vi "Array Parameter Size.vi"() -> ()   [LabVIEW 2020]
uses:
  868a90fa-e97d-4ae1-b623-939be4d37f0a.vi
  d44bdd64-d287-4cd4-98fd-2ffcf2f89dc6.vi
  <userlib>/_NEVSTOP/Communicable State Machine(CSM)/addons/MassData-Parameter/_support/FGV-MassData.vi
  <userlib>/_NEVSTOP/Communicable State Machine(CSM)/addons/MassData-Parameter/CSM MassData Parameter Support.lvlib
panel:
  out "Argument":string
  out "DBL":i32[](array[numeric])
  out "inside 2":i32
  out "inside":i32
  out "outside":i32
  out "unit (ms)":dbl[][](graph)
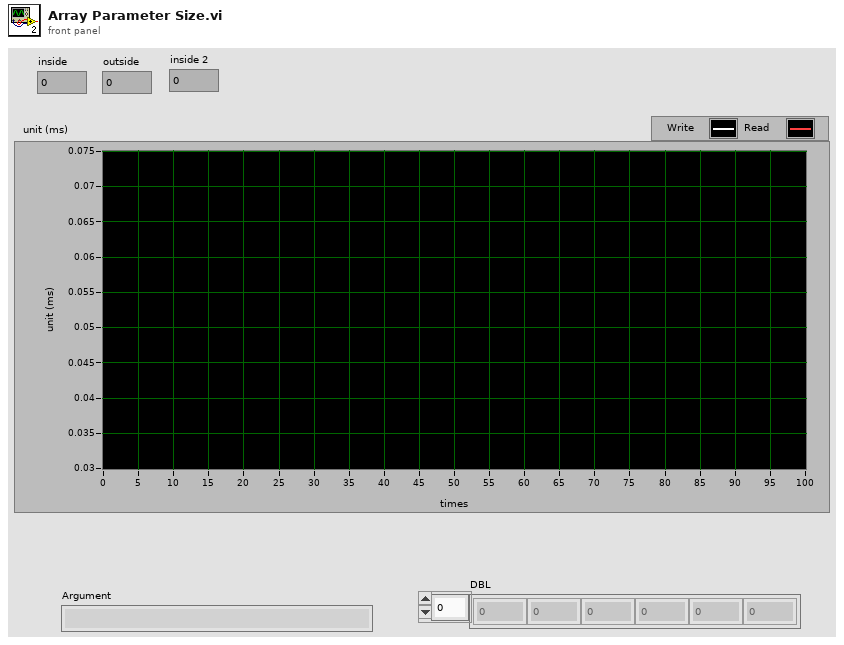
[diagram p1: front panel]
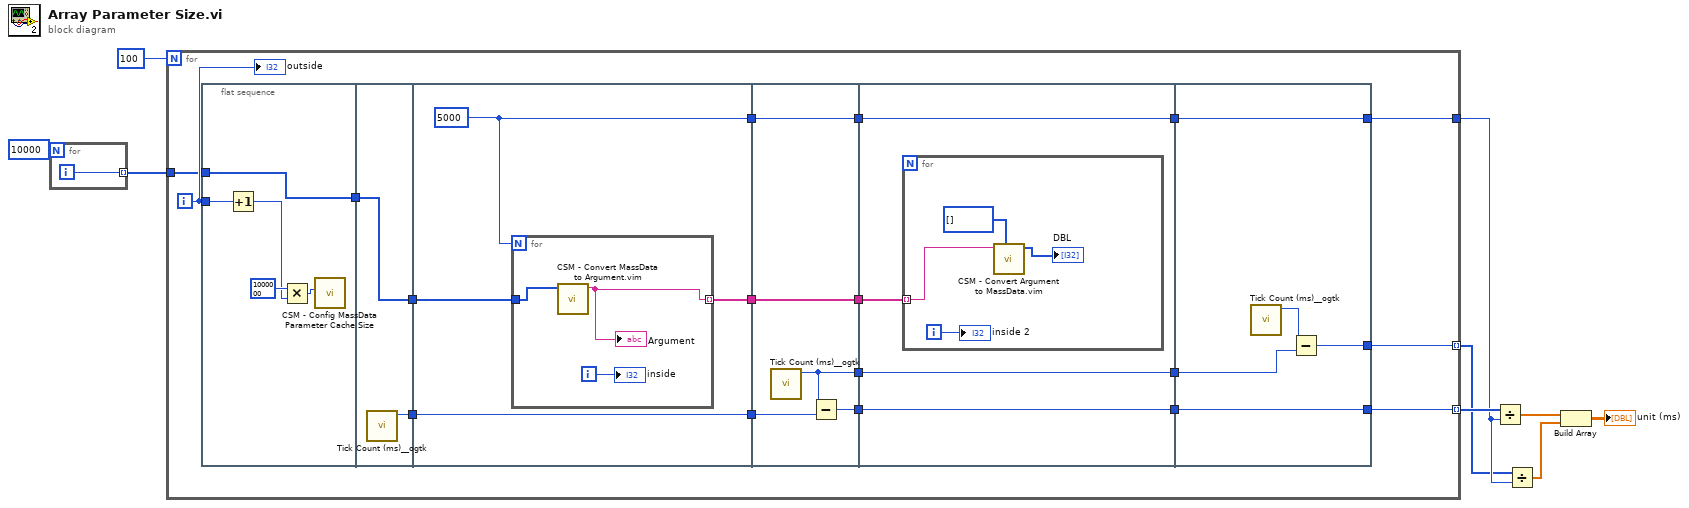
[diagram p0: block diagram]
diagram:
  n1 = for {
    N: 10000 -> [_]
    tunnel: [w10] -> w1 mode=indexing
    i -> [w10]
  }
  n2 = for {
    N: 100 -> [_]
    tunnel: [w26] -> w9 mode=indexing
    tunnel: [w25] -> w5
    tunnel: [w14] -> w4 mode=indexing
    tunnel: w1 -> [w11]
    i -> [w23]
    n3 = flat-sequence {
      tunnel: w23 -> [w31]
      tunnel: [w30] -> w21
      tunnel: w11 -> [w30]
      tunnel: [w35] -> w28
      tunnel: [w34] -> w22
      tunnel: w21 -> [w34]
      tunnel: w28 -> [w39]
      tunnel: [w39] -> w27
      tunnel: [w38] -> w24
      tunnel: w22 -> [w37]
      tunnel: [w36] -> w12
      tunnel: w27 -> [w47]
      tunnel: w24 -> [w45]
      tunnel: [w46] -> w20
      tunnel: [w45] -> w19
      tunnel: [w44] -> w15
      tunnel: [w43] -> w13
      tunnel: w12 -> [w43]
      tunnel: w20 -> [w51]
      tunnel: w19 -> [w50]
      tunnel: [w51] -> w18
      tunnel: [w50] -> w17
      tunnel: [w49] -> w16
      tunnel: w15 -> [w49]
      tunnel: w13 -> [w48]
      tunnel: [w59] -> w25
      tunnel: [w60] -> w26
      tunnel: w18 -> [w60]
      tunnel: w17 -> [w59]
      tunnel: w16 -> [w57]
      tunnel: [w56] -> w14
      frame #0 {
        n4 = Increment(x=w31) -> (x+1=w29:i32)
        n5 = Multiply(x=1000000 ("size(1M)"), y=w29) -> (x*y=w32:i32)
        n6 = call <userlib>:"CSM - Config MassData Parameter Cache Size.vi"("size(1M)"=w32) -> ()  [unwired: 10 in, 1 out]
      }
      frame #1 {
        n7 = call <userlib>:"Tick Count (ms)__ogtk.vi"() -> ("millisecond timer value"=w35:u32)  [unwired: 10 in, 1 out]
      }
      frame #2 {
        w38 = 5000
        n8 = for {
          N: w38 -> [_]
          tunnel: w37 -> [w41]
          tunnel: [w40] -> w36 mode=indexing
          i -> [w42]
          n9 = call "CSM - Convert MassData to Argument.vim"("DBL"=w41) -> ("MassData Argument"=w40:string)  [unwired: 7 in, 1 out]
          "Argument" <- w40
          "inside" <- w42
        }
      }
      frame #3 {
        n10 = call <userlib>:"Tick Count (ms)__ogtk.vi"() -> ("millisecond timer value"=w44:u32)  [unwired: 10 in, 1 out]
        n11 = Subtract(x=w44, y=w47) -> (x-y=w46:u32)
      }
      frame #4 {
        n12 = for {
          tunnel: w48 -> [w53] mode=indexing
          i -> [w55]
          n13 = call "CSM - Convert Argument to MassData.vim"("Type"=i32[] [], "MassData Argument"=w53) -> ("Data"=→"DBL":i32[])  [unwired: 6 in, 1 out]
          "inside 2" <- w55
        }
      }
      frame #5 {
        n14 = call <userlib>:"Tick Count (ms)__ogtk.vi"() -> ("millisecond timer value"=w58:u32)  [unwired: 10 in, 1 out]
        n15 = Subtract(x=w58, y=w57) -> (x-y=w56:u32)
      }
    }
    "outside" <- w23
  }
  n16 = Divide(x=w9, y=w5) -> (x/y=w6:dbl[])
  n17 = Divide(x=w4, y=w5) -> (x/y=w3:dbl[])
  n18 = Build Array(w6, w3) -> (→"unit (ms)":dbl[][])
